vi "CryoCooler Generate HK List.vi"(11 "Num Cryos":i32) -> (2 "Channel Names":string[](array[string])=["Telescope RA", "Telescope DEC", "Telescope Moving?", "Telescope Status"], 3 "Channel List":refnum<class "HK Item.lvclass">[](array[class]))   [LabVIEW 2024]
uses:
  hk-channel-class/hk-channel-class/HK Item/HK Item.lvclass
  hk-channel-class/hk-channel-class/HK Item/HK Channel Units and Setup.ctl
  hk-channel-class/hk-channel-class/HK Item/HK Channel enum Data Type.ctl
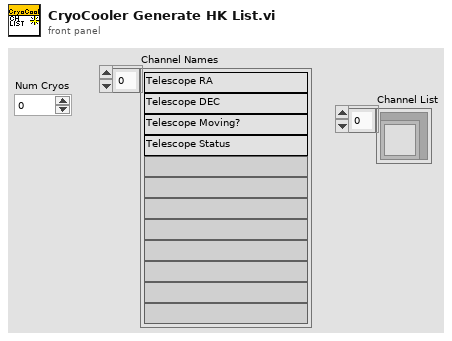
[diagram p1: front panel]
types:
  T1 = typedef "HK Item.lvclass/HK Channel Units and Setup.ctl" = cluster{"Unit Type":string, "Units":string, "Configuration":string, "Digits":i32, "Data Type":T2, "Exponential?":bool, "Source":string}
  T2 = typedef "HK Item.lvclass/HK Channel enum Data Type.ctl" = enum16{"Floating Point", "Integer", "Enum", "String", "Waveform", "File"}
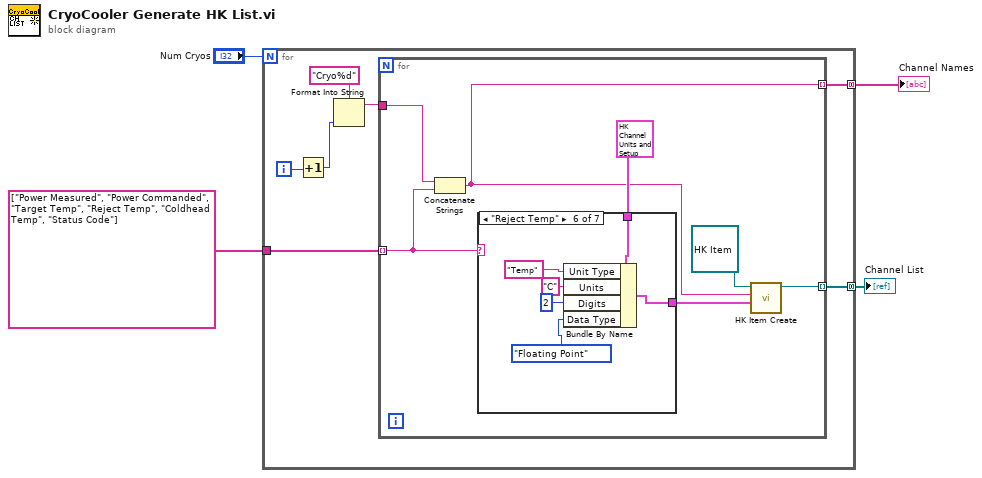
[diagram p0: block diagram]
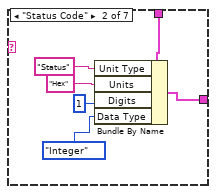
[diagram p3: hidden frame]
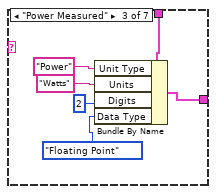
[diagram p4: hidden frame]
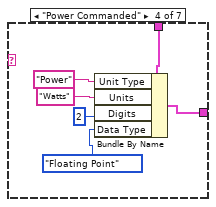
[diagram p5: hidden frame]
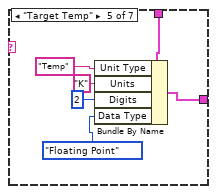
[diagram p6: hidden frame]
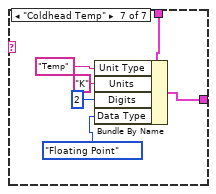
[diagram p7: hidden frame]
diagram:
  n1 = for {
    N: "Num Cryos" -> [_]
    tunnel: string[] ["Power Measured", "Power Commanded", "Target Temp", "Reject Temp", "Coldhead Temp", "Status Code"] -> [w11]
    tunnel: [w10] -> w3 mode=concatenating
    tunnel: [w9] -> w2 mode=concatenating
    i -> [w6]
    n2 = Increment(x=w6) -> (x+1=w5:i32)
    n3 = Format Into String(format string="Cryo%d", w5) -> (resulting string=w8:string)  [unwired: 2 in, 1 out]
    n4 = for {
      tunnel: w11 -> [w13] mode=indexing
      tunnel: [w16] -> w10 mode=indexing
      tunnel: w8 -> [w14]
      tunnel: [w12] -> w9 mode=indexing
      n5 = Concatenate Strings(w14, w13) -> (w12:string)
      n6 = case shown="\"Reject Temp\"" w13 {
        tunnel: T1 {"Unit Type"="", "Units"="", "Configuration"="", "Digits"=3, "Data Type"=enum."Floating Point", "Exponential?"=FALSE, "Source"=""} ("Channel Setup") -> [w19 w25 w31 w37 w43 w49 w55]
        tunnel: [w19 w20 w26 w32 w39 w45 w51] -> w18
        frame "False", Default {
        }
        frame "Status Code" {
          n7 = Bundle By Name(cluster=w25, "Unit Type"="Status", "Units"="Hex", "Digits"=1, "Data Type"=HK_Channel_enum_Data_Type."Integer") -> (w20:T1)
        }
        frame "Power Measured" {
          n8 = Bundle By Name(cluster=w31, "Unit Type"="Power", "Units"="Watts", "Digits"=2, "Data Type"=HK_Channel_enum_Data_Type."Floating Point") -> (w26:T1)
        }
        frame "Power Commanded" {
          n9 = Bundle By Name(cluster=w37, "Unit Type"="Power", "Units"="Watts", "Digits"=2, "Data Type"=HK_Channel_enum_Data_Type."Floating Point") -> (w32:T1)
        }
        frame "Target Temp" {
          n10 = Bundle By Name(cluster=w43, "Unit Type"="Temp", "Units"="K", "Digits"=2, "Data Type"=HK_Channel_enum_Data_Type."Floating Point") -> (w39:T1)
        }
        frame "Reject Temp" {
          n11 = Bundle By Name(cluster=w49, "Unit Type"="Temp", "Units"="C", "Digits"=2, "Data Type"=HK_Channel_enum_Data_Type."Floating Point") -> (w45:T1)
        }
        frame "Coldhead Temp" {
          n12 = Bundle By Name(cluster=w55, "Unit Type"="Temp", "Units"="K", "Digits"=2, "Data Type"=HK_Channel_enum_Data_Type."Floating Point") -> (w51:T1)
        }
      }
      n13 = call-dynamic "HK Item Create.vi"("Channel Setup"=w18, "Name"=w12, "HK Item in"=refnum<class "HK Item.lvclass"> refnum) -> ("HK Item out"=w16:refnum<class "HK Item.lvclass">)  [unwired: 7 in, 1 out]
    }
  }
  "Channel List" <- w3
  "Channel Names" <- w2
